vi "Compare_Costs_(101)_F()_Rearrange_Indices-1.vi"(5 "[IN] Cost functions":i8[](array[numeric]), 6 "[IN] # of Longest track\nInside the Tracks Group":i32, 7 "[IN] Subtracks":T1(array[cluster])) -> (2 "[OUT] Indicies of sub\ntracks for transforma\ntion (resolving)":i32[](array[numeric]))   [LabVIEW 2013]
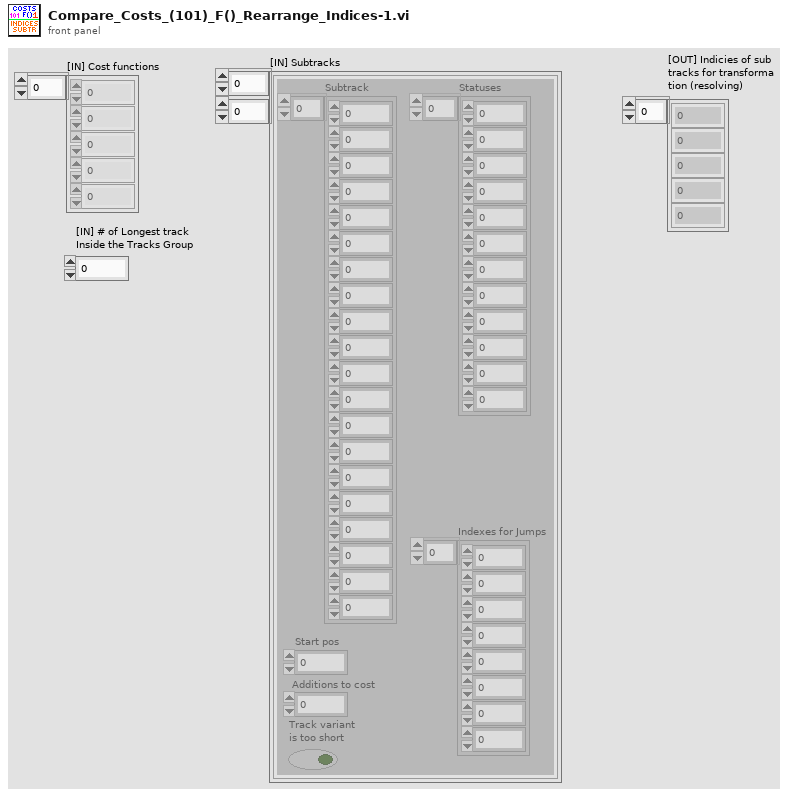
[diagram p1: front panel]
types:
  T1 = cluster{"Subtrack":dbl[], "Statuses":i16[], "Start pos":i32, "Additions to cost":i32, "Track variant \nis too short":bool, "Indexes for Jumps":i32[]}[][]
  T2 = cluster{"Subtrack":dbl[], "Statuses":i16[], "Start pos":i32, "Additions to cost":i32, "Track variant \nis too short":bool, "Indexes for Jumps":i32[]}
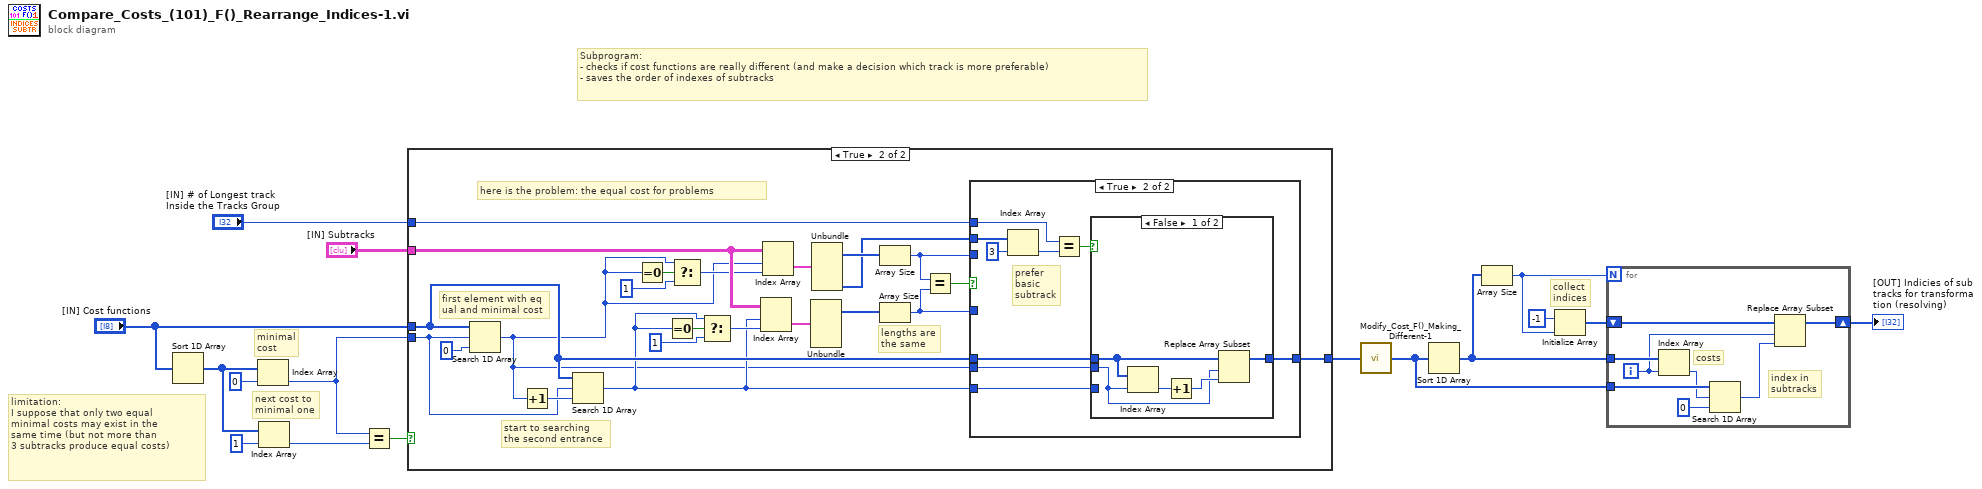
[diagram p0: block diagram]
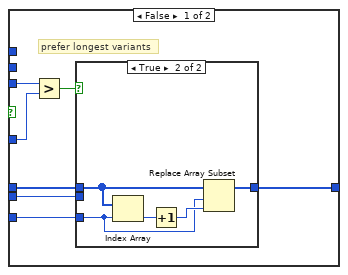
[diagram p3: hidden frame]
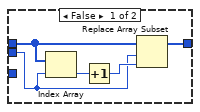
[diagram p4: hidden frame]
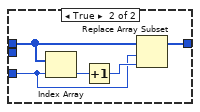
[diagram p5: hidden frame]
diagram:
  # "collect\nindices"
  # "limitation: \nI suppose that only two equal\nminimal costs may exist in the \nsame time (but not more than\n3 subtracks produce equal costs)"
  # "next cost to \nminimal one"
  # "minimal\ncost"
  # "Subprogram:\n- checks if cost functions are really different (and make a decision which track is more preferable)\n- saves the order of indexes of subtracks"
  n1 = Sort 1D Array(array="[IN] Cost functions") -> (sorted array=w11:i8[])
  n2 = Index Array(array=w11, index=0) -> (element=w10:i8)
  n3 = Index Array(array=w11, index=1) -> (element=w14:i8)
  n4 = Equal?(x=w10, y=w14) -> (x = y?=w13:bool)
  n5 = case shown="True" w13 {
    tunnel: "[IN] Subtracks" -> [_ w36]
    tunnel: "[IN] Cost functions" -> [w17 w29]
    tunnel: w10 -> [_ w38]
    tunnel: "[IN] # of Longest track\nInside the Tracks Group" -> [_ w31]
    tunnel: [w17 w26] -> w2
    frame False {
    }
    frame True {
      # "lengths are\nthe same"
      # "start to searching\nthe second entrance"
      # "first element with eq\nual and minimal cost"
      # "here is the problem: the equal cost for problems"
      n6 = Search 1D Array(1D array=w29, element=w38, start index (0)=0) -> (index of element=w18:i32)
      n7 = Increment(x=w18) -> (x+1=w39:i32)
      n8 = Search 1D Array(1D array=w29, element=w38, start index (0)=w39) -> (index of element=w20:i32)
      n9 = Equal To 0?(x=w18) -> (x = 0?=w25:bool)
      n10 = Equal To 0?(x=w20) -> (x = 0?=w23:bool)
      n11 = Select(t=w18, s=w25, f=1) -> (s? t:f=w19:i32)
      n12 = Select(t=w20, s=w23, f=1) -> (s? t:f=w21:i32)
      n13 = Index Array(array=w36, index (row)=w20, index (col)=w21) -> (element=w35:T2)
      n14 = Index Array(array=w36, index (row)=w18, index (col)=w19) -> (element=w37:T2)
      n15 = Unbundle(w35) -> ("Statuses"=w33:i16[])  [unwired: 5 out]
      n16 = Unbundle(w37) -> ("Statuses"=w34:i16[], "Indexes for Jumps"=w30:i32[])  [unwired: 4 out]
      n17 = Array Size(array=w34) -> (size(s)=w28:i32)
      n18 = Array Size(array=w33) -> (size(s)=w27:i32)
      n19 = Equal?(x=w28, y=w27) -> (x = y?=w32:bool)
      n20 = case shown="True" w32 {
        tunnel: w31 -> [_ w64]
        tunnel: w30 -> [_ w66]
        tunnel: w29 -> [w44 w61]
        tunnel: [w41 w60] -> w26
        tunnel: w20 -> [w43 w59]
        tunnel: w18 -> [w42 w58]
        tunnel: w28 -> [w47 _]
        tunnel: w27 -> [w46 _]
        frame False {
          # "prefer longest variants"
          n21 = Greater?(x=w47, y=w46) -> (0:w45:bool)
          n22 = case shown="True" w45 {
            tunnel: w44 -> [w50 w56]
            tunnel: [w49 w54] -> w41
            tunnel: w43 -> [_ w53]
            tunnel: w42 -> [w48 _]
            frame False {
              n23 = Index Array(array=w50, index=w48) -> (element=w52:i8)
              n24 = Increment(x=w52) -> (x+1=w51:i8)
              n25 = Replace Array Subset(array=w50, new element=w51, index=w48) -> (w49:i8[])
            }
            frame True {
              n26 = Index Array(array=w56, index=w53) -> (element=w57:i8)
              n27 = Increment(x=w57) -> (x+1=w55:i8)
              n28 = Replace Array Subset(array=w56, new element=w55, index=w53) -> (w54:i8[])
            }
          }
        }
        frame True {
          # "prefer \nbasic \nsubtrack"
          n29 = Index Array(array=w66, index=3) -> (element=w63:i32)
          n30 = Equal?(x=w64, y=w63) -> (x = y?=w62:bool)
          n31 = case shown="False" w62 {
            tunnel: w61 -> [w69 w75]
            tunnel: [w68 w73] -> w60
            tunnel: w59 -> [_ w72]
            tunnel: w58 -> [w67 _]
            frame False {
              n32 = Index Array(array=w69, index=w67) -> (element=w71:i8)
              n33 = Increment(x=w71) -> (x+1=w70:i8)
              n34 = Replace Array Subset(array=w69, new element=w70, index=w67) -> (w68:i8[])
            }
            frame True {
              n35 = Index Array(array=w75, index=w72) -> (element=w76:i8)
              n36 = Increment(x=w76) -> (x+1=w74:i8)
              n37 = Replace Array Subset(array=w75, new element=w74, index=w72) -> (w73:i8[])
            }
          }
        }
      }
    }
  }
  n38 = call "Modify_Cost_F()_Making_Different-1.vi"("[IN] Cost functions"=w2) -> ("[OUT] Cost functions"=w1:i8[])
  n39 = Sort 1D Array(array=w1) -> (sorted array=w4:i8[])
  n40 = Array Size(array=w4) -> (size(s)=w6:i32)
  n41 = Initialize Array(-1 ("index"), w6) -> (w5:i32[])
  n42 = for {
    N: w6 -> [_]
    shift-right: [w78] -> w3
    shift-left: w5 -> [w80]
    tunnel: w4 -> [w84]
    tunnel: w1 -> [w83]
    i -> [w77]
    # "index in\nsubtracks"
    # "costs"
    n43 = Index Array(array=w84, index=w77) -> (element=w82:i8)
    n44 = Search 1D Array(1D array=w83, element=w82, start index (0)=0) -> (index of element=w79:i32)
    n45 = Replace Array Subset(array=w80, new element=w79, index=w77) -> (w78:i32[])
  }
  "[OUT] Indicies of sub\ntracks for transforma\ntion (resolving)" <- w3
